vi "Generate Contraction Values.vi"(3 "Height":u32) -> (0 "Heights":dbl[](array[numeric]), 1 "Origins":cluster{i32, dbl}[](array[cluster]))   [LabVIEW 2013]
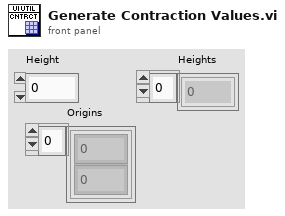
[diagram p1: front panel]
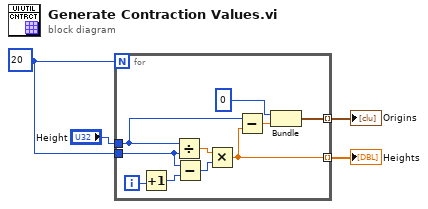
[diagram p0: block diagram]
diagram:
  w4 = 20
  n1 = for {
    N: w4 -> [_]
    tunnel: w4 -> [w5]
    tunnel: "Height" -> [w11]
    tunnel: [w9] -> w2 mode=indexing
    tunnel: [w8] -> w1 mode=indexing
    i -> [w10]
    n2 = Increment(x=w10) -> (x+1=w6:i32)
    n3 = Divide(x=w11, y=w5) -> (x/y=w14:dbl)
    n4 = Subtract(x=w5, y=w6) -> (x-y=w7:i32)
    n5 = Multiply(x=w14, y=w7) -> (x*y=w8:dbl)
    n6 = Subtract(x=w11, y=w8) -> (x-y=w12:dbl)
    n7 = Bundle(0, w12) -> (w9:cluster{i32, dbl})  [unwired: 1 in]
  }
  "Origins" <- w2
  "Heights" <- w1
